vi "Error - Fire Error.vi"(7 "ErrorType":T1, 8 "error in (no error)":errorcluster, 11 "View Model":T2) -> (0 "error out":errorcluster, 3 "View Model":T2)   [LabVIEW 2017]
doc: "Generate an user event which signals about occurred error."
uses:
  View Model/Controls/View Model.ctl
  View Model/Controls/Shared Model.ctl
  Controls/Error Model.ctl
  Controls/Error Event.ctl
  Controls/Error Type.ctl
  Controller/Controls/Controller Model.ctl
  Controller/Controls/Controller Event.ctl
  Controller/Controls/Controller Command.ctl
  Controller/Controls/Controller Overhead.ctl
  Real-Time/RT Status.ctl
  Real-Time/RT Loop Status.ctl
  Controller/Controls/Controller NStream.ctl
  Controller/Controls/Controller DAQ Data.ctl
  TDMS Logger/Controls/TDMS Model.ctl
  TDMS Logger/Controls/TDMS Event.ctl
  TDMS Logger/Controls/TDMS Command.ctl
  TDMS Logger/Controls/TDMS Overhead.ctl
  TDMS Logger/Controls/TDMS ChanNames.ctl
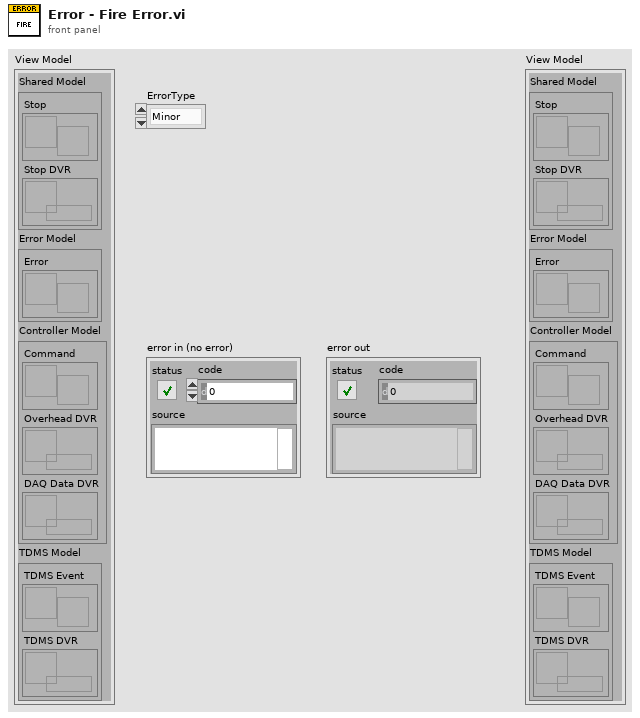
[diagram p1: front panel]
types:
  T1 = typedef "Error Type.ctl" = enum16{"Minor", "Critical"}
  T2 = typedef "View Model.ctl" = cluster{"Shared Model":T3, "Error Model":T4, "Controller Model":T5, "TDMS Model":T6}
  T3 = typedef "Shared Model.ctl" = cluster{"Stop":refnum<user-event>, "Stop DVR":refnum<data-value>}
  T4 = typedef "Error Model.ctl" = cluster{"Error":refnum<user-event>}
  T5 = typedef "Controller Model.ctl" = cluster{"Command":refnum<user-event>, "Overhead DVR":refnum<data-value>, "DAQ Data DVR":refnum<data-value>}
  T6 = typedef "TDMS Model.ctl" = cluster{"TDMS Event":refnum<user-event>, "TDMS DVR":refnum<data-value>}
  T7 = typedef "Error Event.ctl" = cluster{"ErrorType":T1, "error in":errorcluster}
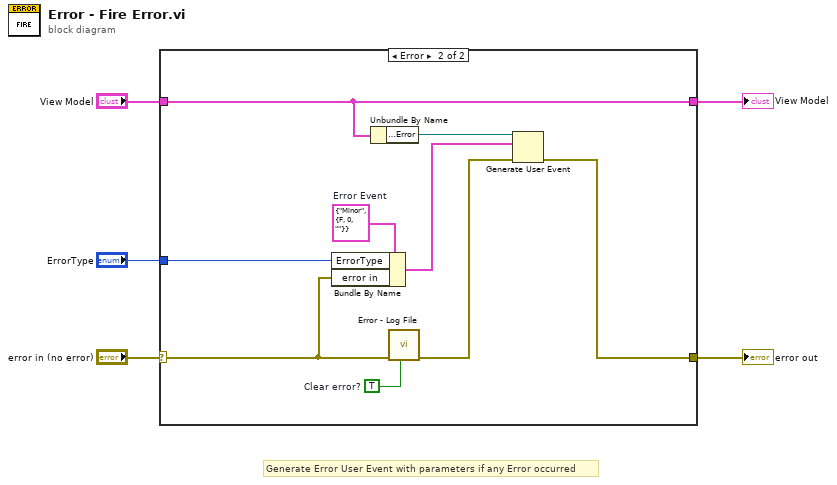
[diagram p0: block diagram]
diagram:
  # "Generate Error User Event with parameters if any Error occurred"
  n1 = case shown="Error" "error in (no error)" {
    selector: "error in (no error)" -> [w7 w10]
    tunnel: [w7 w11] -> w4
    tunnel: "View Model" -> [w6 w14]
    tunnel: [w6 w14] -> w2
    tunnel: "ErrorType" -> [_ w15]
    frame No Error {
    }
    frame Error {
      w8 = TRUE  # Clear error?
      w16 = T7 {"ErrorType"=enum."Minor", "error in"={"status"=FALSE, "code"=0, "source"=""}}  # Error Event
      n2 = Bundle By Name(cluster=w16, "ErrorType"=w15, "error in"=w10) -> (w12:T7)
      n3 = Unbundle By Name(w14) -> ("Error Model.Error"=w13:refnum<user-event>)
      n4 = call "Error - Log File.vi"("Clear error?"=w8, "error in"=w10) -> ("error out"=w9:errorcluster)  [unwired: 9 in]
      n5 = Generate User Event(user event=w13, event data cluster=w12, error in=w9) -> (error out=w11:errorcluster)  [unwired: 1 in, 1 out]
    }
  }
  "View Model" <- w2
  "error out" <- w4
